vi "Batch Dataset Store.vi"(8 "error in":errorcluster, 9 "Data":dbl[][](array[numeric]), 10 "Dataset Source":T1, 11 "Transactions":string[](array[string])) -> (0 "error out":errorcluster)   [LabVIEW 2013]
uses:
  Transactions/Dataset Source.ctl
  Data Access Objects/Metadata/DAO Actions.ctl
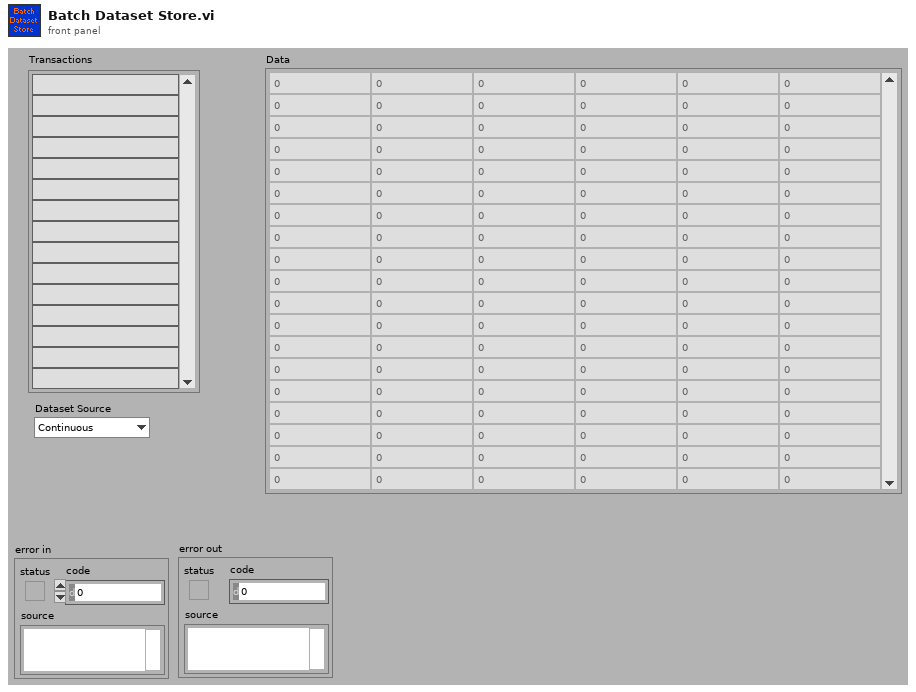
[diagram p1: front panel]
types:
  T1 = typedef "Dataset Source.ctl" = enum16{"Continuous", "Hold", "ED", "Volts", "Offsets", "Increments"}
  T2 = typedef "DAO Actions.ctl" = enum16{"Init", "Get", "Set"}
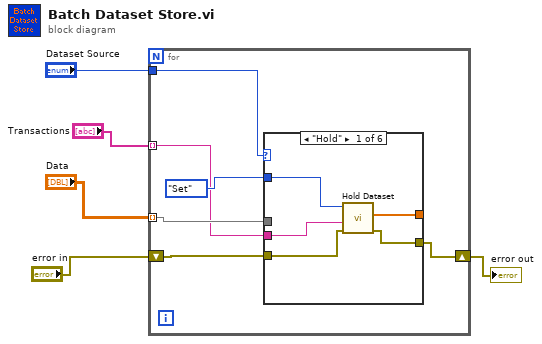
[diagram p0: block diagram]
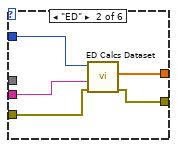
[diagram p2: hidden frame]
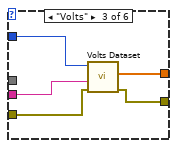
[diagram p3: hidden frame]
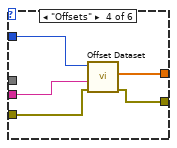
[diagram p4: hidden frame]
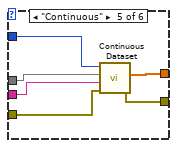
[diagram p5: hidden frame]
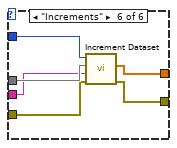
[diagram p6: hidden frame]
diagram:
  n1 = for {
    shift-right: [w7] -> w3
    shift-left: "error in" -> [w9]
    tunnel: "Transactions" -> [w8] mode=indexing
    tunnel: "Data" -> [w10] mode=indexing
    tunnel: "Dataset Source" -> [w6]
    n2 = case shown="\"Hold\"" w6 {
      tunnel: [w16 w21 w26 w31 w37 w41] -> _
      tunnel: DAO_Actions."Set" ("DAO Actions") -> [w15 w20 w25 w30 w36 w43]
      tunnel: [w14 w19 w24 w29 w35 w39] -> w7
      tunnel: w9 -> [w13 w18 w23 w28 w34 w40]
      tunnel: w8 -> [w12 w17 w22 w27 w33 w38]
      tunnel: w10 -> [_ _ _ _ w32 w42]
      frame "Hold" {
        n3 = call "Hold Dataset.vi"("error in (no error)"=w13, "Group ID"=w12, "DAO Actions"=w15) -> ("error out"=w14:errorcluster, "Data Out"=w16:dbl[])  [unwired: 7 in]
      }
      frame "ED" {
        n4 = call "ED Calcs Dataset.vi"("error in (no error)"=w18, "Group ID"=w17, "DAO Actions"=w20) -> ("error out"=w19:errorcluster, "Data Out"=w21:dbl[])  [unwired: 7 in]
      }
      frame "Volts" {
        n5 = call "Volts Dataset.vi"("error in (no error)"=w23, "Group ID"=w22, "DAO Actions"=w25) -> ("error out"=w24:errorcluster, "Data Out"=w26:dbl[])  [unwired: 7 in]
      }
      frame "Offsets" {
        n6 = call "Offset Dataset.vi"("error in (no error)"=w28, "Group ID"=w27, "DAO Actions"=w30) -> ("error out"=w29:errorcluster, "Data Out"=w31:dbl[])  [unwired: 7 in]
      }
      frame "Continuous" {
        n7 = call "Continuous Dataset.vi"("error in (no error)"=w34, "Group ID"=w33, "Data In"=w32, "DAO Actions"=w36) -> ("error out"=w35:errorcluster, "Data Out"=w37:dbl[])  [unwired: 6 in]
      }
      frame "Increments" {
        n8 = call "Increment Dataset.vi"("error in (no error)"=w40, "Group ID"=w38, "Data In"=w42, "DAO Actions"=w43) -> ("error out"=w39:errorcluster, "Data Out"=w41:dbl[])  [unwired: 6 in]
      }
    }
  }
  "error out" <- w3
